vi "题1.vi"() -> ()   [LabVIEW 2017]
uses:
  <vilib>/measure/NI_MABase.lvlib
panel:
  out "波形图 2":waveform(dbl)(graph)
  out "波形图":waveform(dbl)(graph)
  in  "布尔":bool
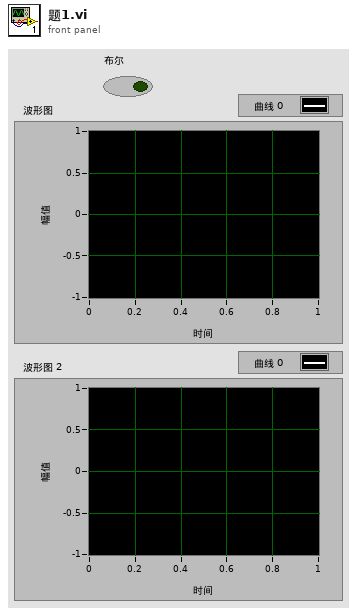
[diagram p1: front panel]
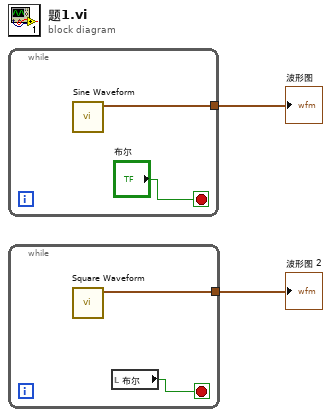
[diagram p0: block diagram]
diagram:
  n1 = while {
    tunnel: [w4] -> w1
    stop <- "布尔" stop-if-true
    n2 = call <vilib>:"Sine Waveform.vi"() -> ("signal out"=w4:waveform(dbl))  [unwired: 10 in, 1 out]
  }
  "波形图" <- w1
  n3 = while {
    tunnel: [w6] -> w2
    stop <- w5 stop-if-true
    n4 = call <vilib>:"Square Waveform.vi"() -> ("signal out"=w6:waveform(dbl))  [unwired: 10 in, 1 out]
    n5 = local read "布尔"() -> (w5:bool)
  }
  "波形图 2" <- w2
